vi "remap tag and channel.vi"(7 "instance id":string, 8 "error in":errorcluster, 9 "tag name":string, 10 "channel":refnum<class "TBM channel.lvclass">, 11 "engine configuration in":refnum<class "engine configuration.lvclass">) -> (0 "error out":errorcluster, 3 "engine configuration out":refnum<class "engine configuration.lvclass">)   [LabVIEW 2013, in "configuration tests.lvlib" / "TEST EDITOR.lvclass"]
uses:
  TEST EDITOR.lvclass
  <vilib>/NI/Module Execution Interface/Engine Configuration/engine configuration.lvclass
  <vilib>/NI/Tag Bus Module Framework/channel/TBM channel.lvclass
  <vilib>/NI/Tag Bus/tag/tag descriptor.lvclass/tag descriptor.ctl
  <vilib>/NI/Tag Bus/tag/write tag name.vi
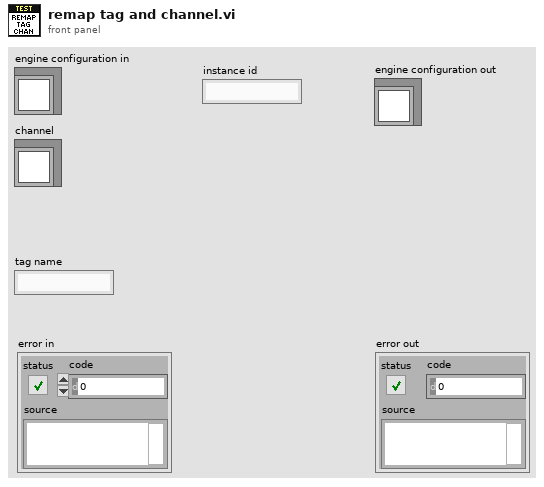
[diagram p1: front panel]
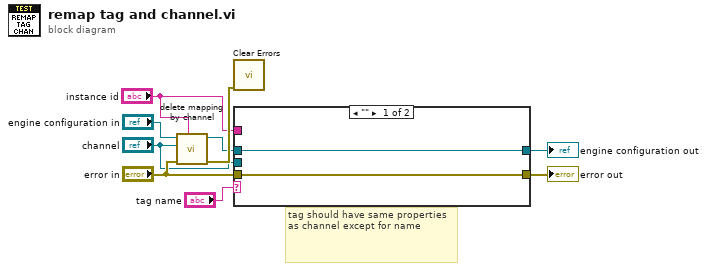
[diagram p0: block diagram]
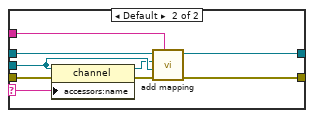
[diagram p2: hidden frame]
diagram:
  # "tag should have same properties as channel except for name"
  n1 = call <vilib>:"delete mapping by channel.vi"("owner ID"="instance id", "error in"="error in", "channel"="channel", "engine configuration in"="engine configuration in") -> ("error out"=w9:errorcluster, "engine configuration out"=w3:refnum<class "engine configuration.lvclass">)  [unwired: 6 in]
  n2 = call <vilib>:"Clear Errors.vi"("error in (no error)"=w9) -> ()  [unwired: 6 in, 1 out]
  n3 = case shown="\"\"" "tag name" {
    selector: "tag name" -> [_ w12]
    tunnel: "error in" -> [w10 w20]
    tunnel: "instance id" -> [_ w19]
    tunnel: [w10 w18] -> w6
    tunnel: [w11 w17] -> w5
    tunnel: "channel" -> [_ w15]
    tunnel: w3 -> [w11 w13]
    frame "" {
    }
    frame Default {
      n4 = property class="channel"(reference=w15, error in=w20, "accessors:name"=w12) -> (reference out=w14:refnum<class "TBM channel.lvclass">, error out=w16:errorcluster)
      n5 = call <vilib>:"add mapping.vi"("owner ID"=w19, "error in"=w16, "channel"=w15, "tag descriptor"=w14, "engine configuration"=w13) -> ("error out"=w18:errorcluster, "engine configuration out"=w17:refnum<class "engine configuration.lvclass">)  [unwired: 5 in]
    }
  }
  "error out" <- w6
  "engine configuration out" <- w5
